vi "Update Origin.vi"(8 "error in (no error)":errorcluster, 10 "Origin":cluster{"X":dbl, "Y":dbl, "R":dbl}, 11 "Yaml Model in":refnum<class "Yaml Model.lvclass">) -> (0 "error out":errorcluster, 3 "Yaml Model out":refnum<class "Yaml Model.lvclass">)   [LabVIEW 2020, in "Yaml Model.lvlib" / "Yaml Model.lvclass"]
uses:
  Yaml Model.lvclass
  Yaml Model.lvclass/Yaml Model.ctl
panel:
  # "NOTICE -- YOU MUST LEAVE THIS NOTICE IN PLACE.\n\nCopyright (c) 2017, LIANG LIU Shawn.Liu.cn@gmail.com\nAll rights reserved.\n\nRedistribution and use in source and binary forms, with or without modification, are permitted provided that the following conditions are met:\n-Redistributions of source code must retain the above copyright notice, this list of conditions and the following disclaimer.\n-Redistributions in binary form must reproduce the above copyright notice, this list of conditions and the following disclaimer in the documentation and/or other materials provided with the distribution.\n-Neither the name of the eLp nor the names of its contributors may be used to endorse or promote products derived from this software without specific prior written permission.\n\nTHIS SOFTWARE IS PROVIDED BY THE COPYRIGHT HOLDERS AND CONTRIBUTORS \"AS IS\" AND ANY EXPRESS OR IMPLIED WARRANTIES, INCLUDING, BUT NOT LIMITED TO, THE IMPLIED WARRANTIES OF MERCHANTABILITY AND FITNESS FOR A PARTICULAR PURPOSE ARE DISCLAIMED. IN NO EVENT SHALL THE COPYRIGHT HOLDER OR CONTRIBUTORS BE LIABLE FOR ANY DIRECT, INDIRECT, INCIDENTAL, SPECIAL, EXEMPLARY, OR CONSEQUENTIAL DAMAGES (INCLUDING, BUT NOT LIMITED TO, PROCUREMENT OF SUBSTITUTE GOODS OR SERVICES; LOSS OF USE, DATA, OR PROFITS; OR BUSINESS INTERRUPTION) HOWEVER CAUSED AND ON ANY THEORY OF LIABILITY, WHETHER IN CONTRACT, STRICT LIABILITY, OR TORT (INCLUDING NEGLIGENCE OR OTHERWISE) ARISING IN ANY WAY OUT OF THE USE OF THIS SOFTWARE, EVEN IF ADVISED OF THE POSSIBILITY OF SUCH DAMAGE."
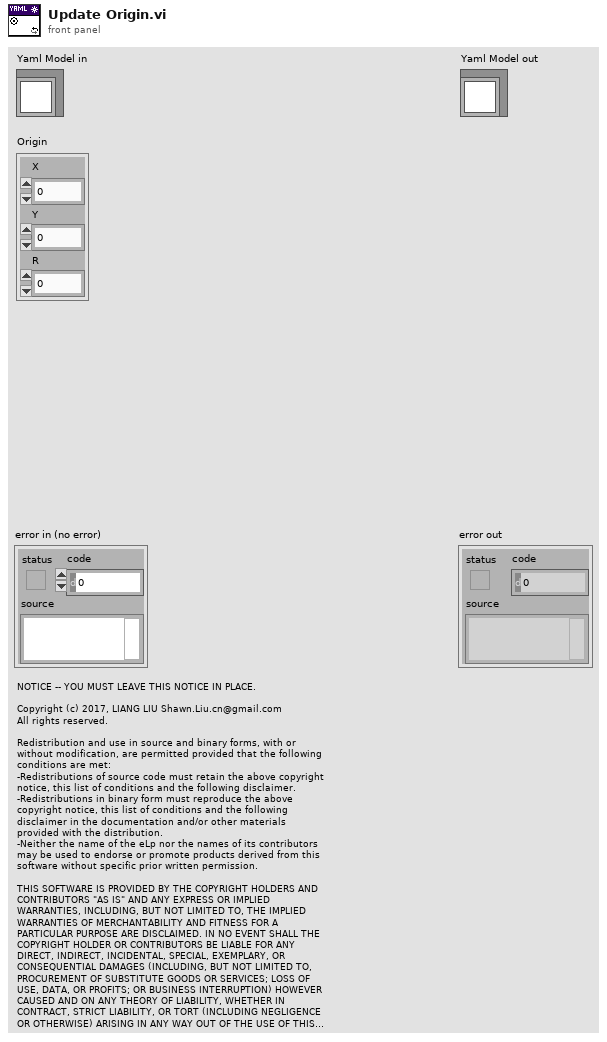
[diagram p1: front panel]
types:
  T1 = enum8{"Enabled", "Disabled", "Disabled and Grayed Out"}
  T2 = cluster{"Image":string, "Resolution":dbl, "Origin":cluster{"X":dbl, "Y":dbl, "R":dbl}, "Occupied Thresh":dbl, "Free Thresh":dbl, "Negate":bool}
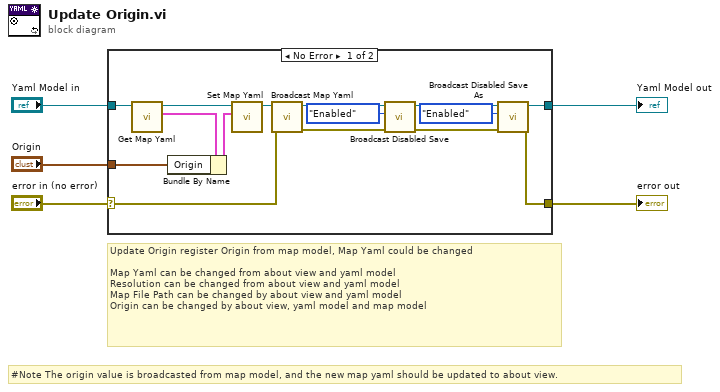
[diagram p0: block diagram]
diagram:
  # "#Note The origin value is broadcasted from map model, and the new map yaml should be updated to about view."
  # "Update Origin register Origin from map model, Map Yaml could be changed\n\nMap Yaml can be changed from about view and yaml model\nResolution can be changed from about view and yaml model\nMap File Path can be changed by about view and yaml model\nOrigin can be changed by about view, yaml model and map model"
  n1 = case shown="No Error" "error in (no error)" {
    selector: "error in (no error)" -> [w20 w22]
    tunnel: "Yaml Model in" -> [w19 w21]
    tunnel: [w18 w21] -> w3
    tunnel: [w17 w22] -> w2
    tunnel: "Origin" -> [w16 _]
    frame No Error {
      n2 = call "Get Map Yaml.vi"("Yaml Model in"=w19) -> ("Map Yaml"=w9:T2, "Yaml Model out"=w10:refnum<class "Yaml Model.lvclass">)  [unwired: 9 in]
      n3 = Bundle By Name(cluster=w9, "Origin"=w16) -> (w8:T2)
      n4 = call "Set Map Yaml.vi"("Map Yaml"=w8, "Yaml Model in"=w10) -> ("Yaml Model out"=w15:refnum<class "Yaml Model.lvclass">)  [unwired: 9 in]
      n5 = call "Broadcast Map Yaml.vi"("error in (no error)"=w20, "Yaml Model in"=w15) -> ("error out"=w6:errorcluster, "Yaml Model out"=w7:refnum<class "Yaml Model.lvclass">)  [unwired: 8 in]
      n6 = call "Broadcast Disabled Save.vi"("error in (no error)"=w6, "Disabled Save"=T1."Enabled", "Yaml Model in"=w7) -> ("error out"=w11:errorcluster, "Yaml Model out"=w14:refnum<class "Yaml Model.lvclass">)  [unwired: 7 in]
      n7 = call "Broadcast Disabled Save As.vi"("error in (no error)"=w11, "Disabled Save As"=T1."Enabled", "Yaml Model in"=w14) -> ("error out"=w17:errorcluster, "Yaml Model out"=w18:refnum<class "Yaml Model.lvclass">)  [unwired: 7 in]
    }
    frame Error {
    }
  }
  "error out" <- w2
  "Yaml Model out" <- w3
